vi "Get_Parameters_Reference.vi"(8 "error in (no error)":errorcluster, 11 "ExampleStateMachine runtime_in":refnum<class "ExampleStateMachine runtime.lvclass">) -> (0 "error out":errorcluster, 2 "Parameters_Reference":dbl[](array[numeric]), 3 "ExampleStateMachine runtime_out":refnum<class "ExampleStateMachine runtime.lvclass">)   [LabVIEW 2017, in "ExampleStateMachine runtime.lvclass"]
uses:
  ExampleStateMachine runtime.lvclass
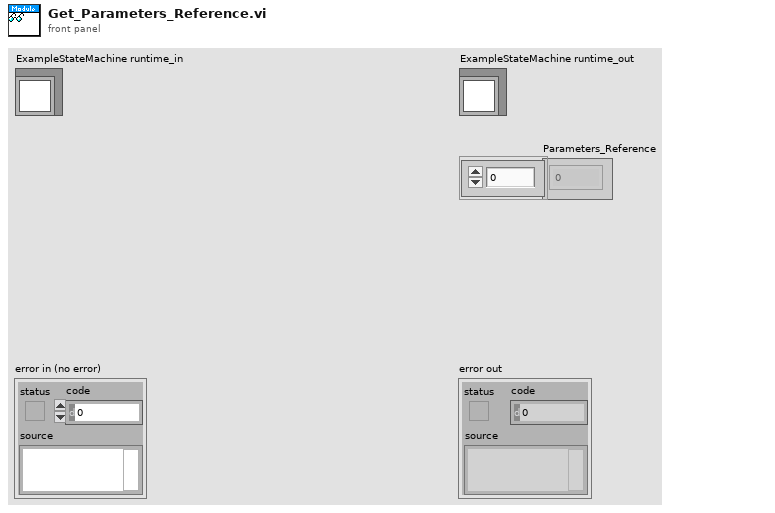
[diagram p1: front panel]
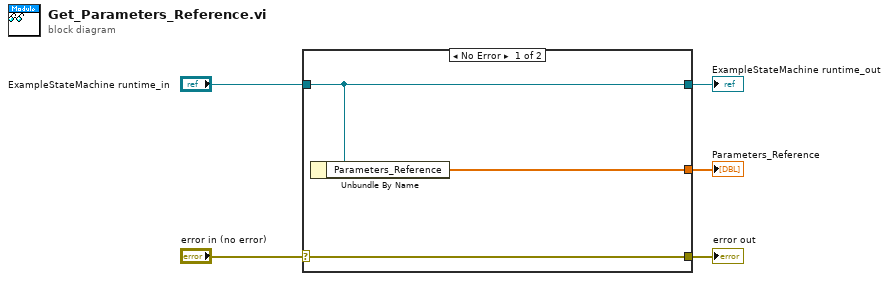
[diagram p0: block diagram]
diagram:
  n1 = case shown="No Error" "error in (no error)" {
    selector: "error in (no error)" -> [w8 w9]
    tunnel: [w8 w9] -> w4
    tunnel: [w7 w10] -> w2
    tunnel: "ExampleStateMachine runtime_in" -> [w7 w10]
    tunnel: [w6 _] -> w1
    frame No Error {
      n2 = Unbundle By Name(w7) -> ("Parameters_Reference"=w6:dbl[])
    }
    frame Error {
    }
  }
  "error out" <- w4
  "ExampleStateMachine runtime_out" <- w2
  "Parameters_Reference" <- w1
